vi "load.vi"() -> ()   [LabVIEW 2012]
uses:
  Global1.vi
  <vilib>/Utility/file.llb/Read From Spreadsheet File (string).vi
panel:
  out "error out":errorcluster
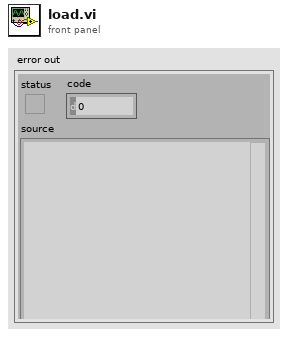
[diagram p1: front panel]
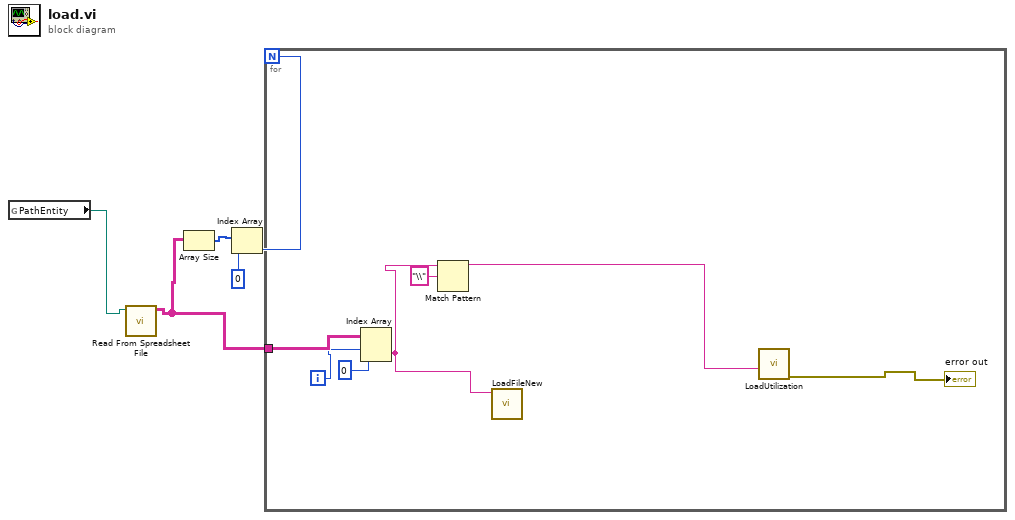
[diagram p0: block diagram]
diagram:
  n1 = global read "Global1.vi" "PathEntity"() -> (w1:path)
  n2 = call-poly <vilib>:"Read From Spreadsheet File.vi"("file path (dialog if empty)"=w1) -> ("all rows"=w2:string[][])  [unwired: 6 in, 4 out]
  n3 = Array Size(array=w2) -> (size(s)=w5:i32[])
  n4 = Index Array(array=w5, index=0) -> (element=w3:i32)
  n5 = for {
    N: w3 -> [_]
    tunnel: w2 -> [w12]
    i -> [w10]
    n6 = Index Array(array=w12, index (row)=w10, index (col)=0 ("disabled index (col)")) -> (element=w8:string)
    n7 = Match Pattern(string=w8, regular expression="\\") -> (before substring=w6:string)  [unwired: 1 in, 3 out]
    n8 = call "LoadFileNew.vi"("folder"=w8) -> ()  [unwired: 9 in, 2 out]
    n9 = call "LoadUtilization.vi"("machine"=w6) -> ("error out"=→"error out":errorcluster)  [unwired: 8 in]
  }
